vi "IMAQdx Add Attribute To Tree.vi"(6 "Display Name":string="Root::AcquisitionControl::AcquisitionStart", 8 "error in":errorcluster, 9 "Value":string="Some string value", 10 "Attribute Name":string="Root::AcquisitionControl::AcquisitionStart", 11 "Attribute Table In":refnum<vi>) -> (0 "error out":errorcluster, 3 "Attribute Table Out":refnum<vi>)   [LabVIEW 2014, in "HGF_VisionTools.lvlib"]
doc: "The Add Attribute To Tree subVI contains the logic to parse the attribute name string and populate the attribute into the Attribute tree control."
uses:
  HGF_VisionTools.lvlib
panel:
  out "Navigate Tree:Get Parent":string
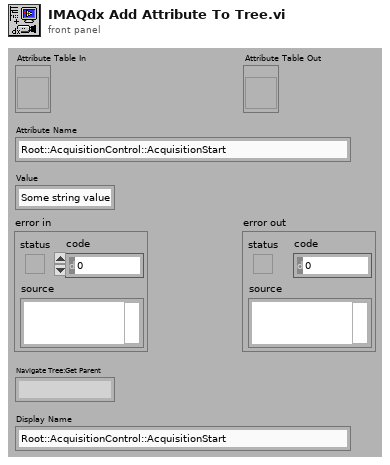
[diagram p1: front panel]
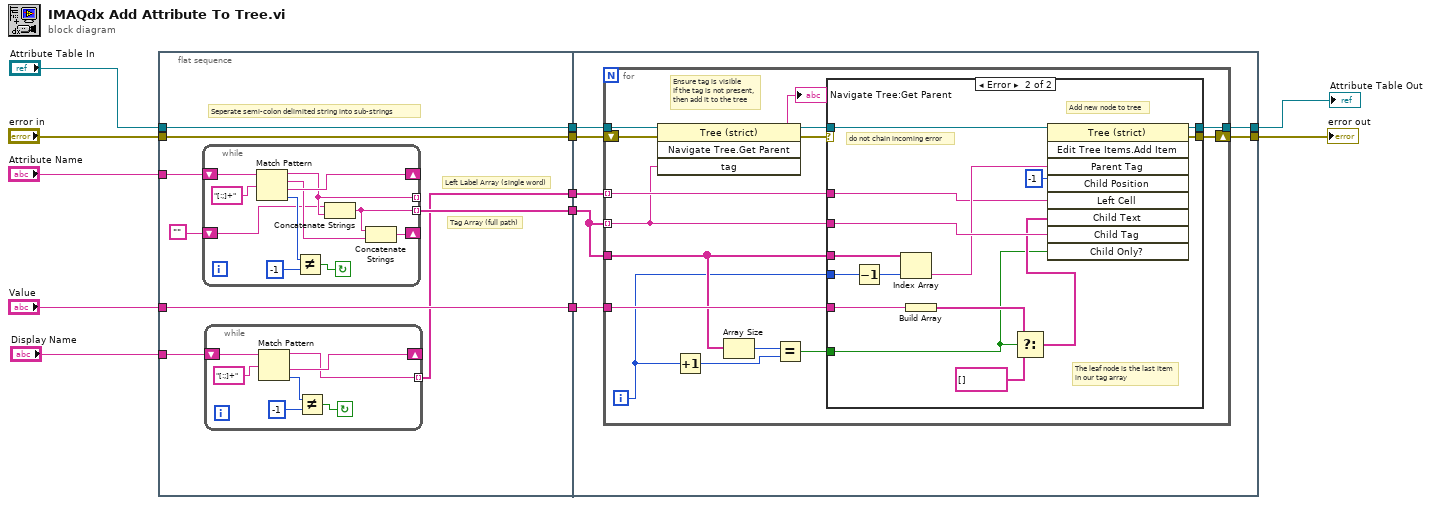
[diagram p0: block diagram]
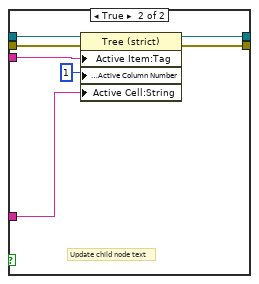
[diagram p3: hidden frame]
diagram:
  n1 = flat-sequence {
    tunnel: "Attribute Name" -> [w19]
    tunnel: [w18] -> w11
    tunnel: [w13] -> w10
    tunnel: "Attribute Table In" -> [w17]
    tunnel: [w17] -> w9
    tunnel: "error in" -> [w16]
    tunnel: [w16] -> w8
    tunnel: "Value" -> [w15]
    tunnel: [w15] -> w4
    tunnel: "Display Name" -> [w14]
    tunnel: w11 -> [w41]
    tunnel: w10 -> [w43]
    tunnel: w9 -> [w45]
    tunnel: w8 -> [w44]
    tunnel: [w42] -> w7
    tunnel: [w40] -> w6
    tunnel: w4 -> [w39]
    frame #0 {
      # "Left Label Array (single word)"
      # "Tag Array (full path)"
      # "Seperate semi-colon delimited string into sub-strings"
      n2 = while {
        shift-right: [w35] -> _
        shift-left: w19 -> [w34]
        tunnel: [w29] -> _ mode=indexing
        shift-right: [w31] -> _
        shift-left: "" -> [w28]
        tunnel: [w32] -> w18 mode=indexing
        stop <- w37 continue-if-true
        n3 = Match Pattern(string=w34, regular expression="[:;]+") -> (before substring=w29:string, match substring=w30:string, after substring=w35:string, offset past match=w33:i32)  [unwired: 1 out]
        n4 = Not Equal?(x=w33, y=-1) -> (x != y?=w37:bool)
        n5 = Concatenate Strings(w28, w29) -> (w32:string)
        n6 = Concatenate Strings(w32, w30) -> (w31:string)
      }
      n7 = while {
        shift-right: [w24] -> _
        shift-left: w14 -> [w23]
        tunnel: [w21] -> w13 mode=indexing
        stop <- w26 continue-if-true
        n8 = Match Pattern(string=w23, regular expression="[:;]+") -> (before substring=w21:string, after substring=w24:string, offset past match=w22:i32)  [unwired: 2 out]
        n9 = Not Equal?(x=w22, y=-1) -> (x != y?=w26:bool)
      }
    }
    frame #1 {
      n10 = for {
        tunnel: w41 -> [w53] mode=indexing
        tunnel: w45 -> [w60]
        tunnel: [w57] -> w40
        tunnel: w43 -> [w54] mode=indexing
        shift-right: [w55] -> w42
        shift-left: w44 -> [w56]
        tunnel: w41 -> [w48]
        tunnel: w39 -> [w52]
        i -> [w47]
        # "Ensure tag is visible\nIf the tag is not present,\nthen add it to the tree"
        n11 = invoke class="Tree (strict)" method="Navigate Tree.Get Parent"(reference=w60, error in=w56, "tag"=w53) -> (reference out=w58:refnum<vi>, error out=w59:errorcluster, "Navigate Tree:Get Parent"=→"Navigate Tree:Get Parent":string)  [unwired: 1 in, 1 out]
        n12 = Increment(x=w47) -> (x+1=w50:i32)
        n13 = Array Size(array=w48) -> (size(s)=w51:i32)
        n14 = Equal?(x=w51, y=w50) -> (x = y?=w49:bool)
        n15 = case shown="Error" w59 {
          selector: w59 -> [w65 _]
          tunnel: w58 -> [w67 w91]
          tunnel: [w66 w90] -> w57
          tunnel: [w64 w88] -> w55
          tunnel: w54 -> [_ w77]
          tunnel: w53 -> [w62 w89]
          tunnel: w48 -> [_ w79]
          tunnel: w52 -> [w61 w83]
          tunnel: w47 -> [_ w82]
          tunnel: w49 -> [w63 w78]
          frame No Error {
            # "This node already exists"
            n16 = case shown="False" w63 {
              tunnel: w67 -> [w69 w76]
              tunnel: [w69 w75] -> w66
              tunnel: w65 -> [w68 w74]
              tunnel: [w68 w73] -> w64
              tunnel: w62 -> [_ w72]
              tunnel: w61 -> [_ w70]
              frame False {
              }
              frame True {
                # "Update child node text"
                n17 = property class="Tree (strict)"(reference=w76, error in=w74, "Active Item:Tag"=w72, "Active Cell:Active Column Number"=1 ("Active Cell Properties:Active Column Number"), "Active Cell:String"=w70) -> (reference out=w75:refnum<vi>, error out=w73:errorcluster)
              }
            }
          }
          frame Error {
            # "Add new node to tree"
            # "The leaf node is the last item\nin our tag array"
            # "do not chain incoming error"
            n18 = Decrement(x=w82) -> (x-1=w84:i32)
            n19 = Index Array(array=w79, index=w84) -> (element=w80:string)
            n20 = Build Array(w83) -> (w85:string[])
            n21 = Select(t=w85, s=w78, f=string[] [] ("t")) -> (s? t:f=w81:string[])
            n22 = invoke class="Tree (strict)" method="Edit Tree Items.Add Item"(reference=w91, "Parent Tag"=w80, "Child Position"=-1, "Left Cell"=w77, "Child Text"=w81, "Child Tag"=w89, "Child Only?"=w78) -> (reference out=w90:refnum<vi>, error out=w88:errorcluster)  [unwired: 2 in, 7 out]
          }
        }
      }
    }
  }
  "error out" <- w7
  "Attribute Table Out" <- w6
